vi "ScanAction.vi"(8 "error in (no error)":errorcluster caption="entrée d'erreur (pas d'erreur)", 9 "IndicePoint":i32, 10 "Dir":bool, 11 "Tools In":refnum<class "AttoANC300.lvclass"> caption="DNL_LabVIEW Object in") -> (0 "error out":errorcluster caption="sortie d'erreur", 2 "ScanParsOut":dbl[](array[numeric]), 3 "Tools Out":refnum<class "AttoANC300.lvclass"> caption="DNL_LabVIEW Object out")   [LabVIEW 2019, in "AttoANC300.lvclass"]
uses:
  AttoANC300.lvclass
  C:/Programmes Labview/LabscanV1A/DevicesClass/BaseDevice/BaseDevice.lvclass
  AttoANC300.lvclass/AttoANC300.ctl
  AttoAMC/ScanActionStates.ctl
  <userlib>/GenProg/WritebyWeakRefNum.vi
  <vilib>/Utility/error.llb/Error Cluster From Error Code.vi
  <vilib>/ErrorRing/Error Ring.xnode
  <userlib>/AMC300/AMC_VIs.lvlib
panel:
  in  "Reactivate":bool
  out "axis":i32
  out "Bkwd":bool
  out "Fwd":bool
  out "Trgt Rng(nm)":dbl
  in  "CtrlLpReact":u32
  out "PosDiff(nm)":dbl
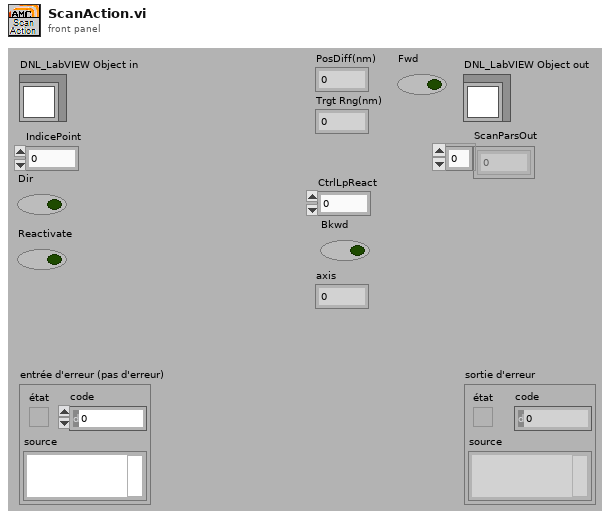
[diagram p1: front panel]
types:
  T1 = typedef "ScanActionStates.ctl" = enum16{"ReadPosDiff", "SetTarget", "WaitMoveDone", "MoveDone", "Timeout", "Ctrl_Loop_React", "Limit_check", "Error"}
  T2 = typedef "AttoANC300.lvclass/AttoANC300_Func.ctl" = enum16{"MotionMon (um)", "VoltDC (V)"}
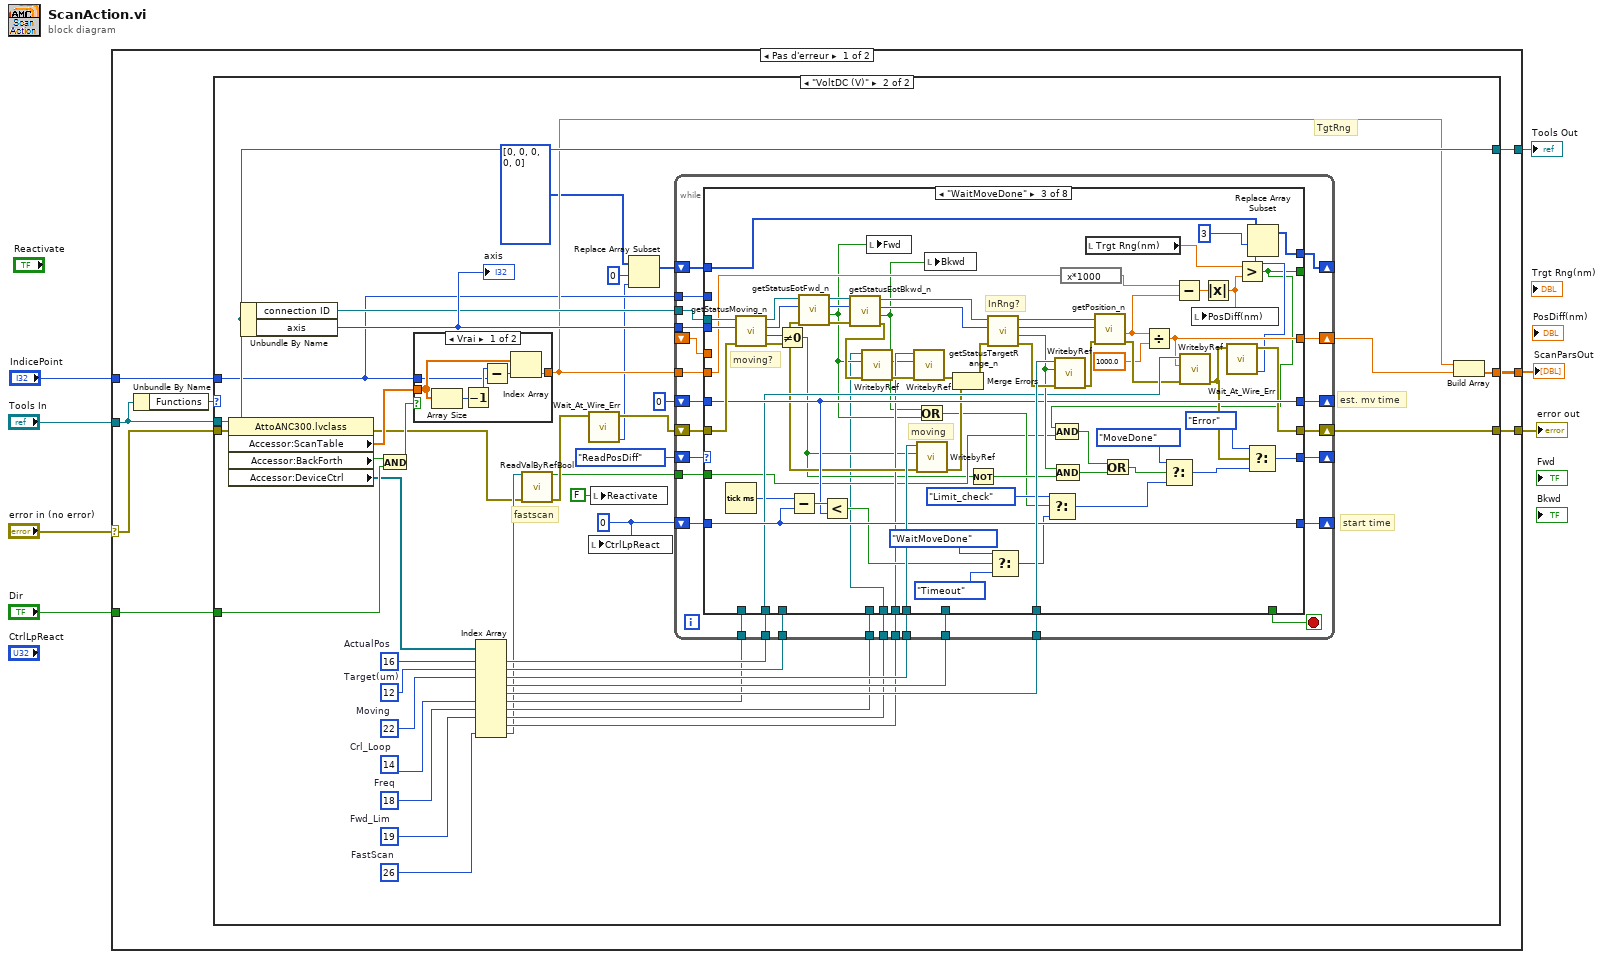
[diagram p0: block diagram]
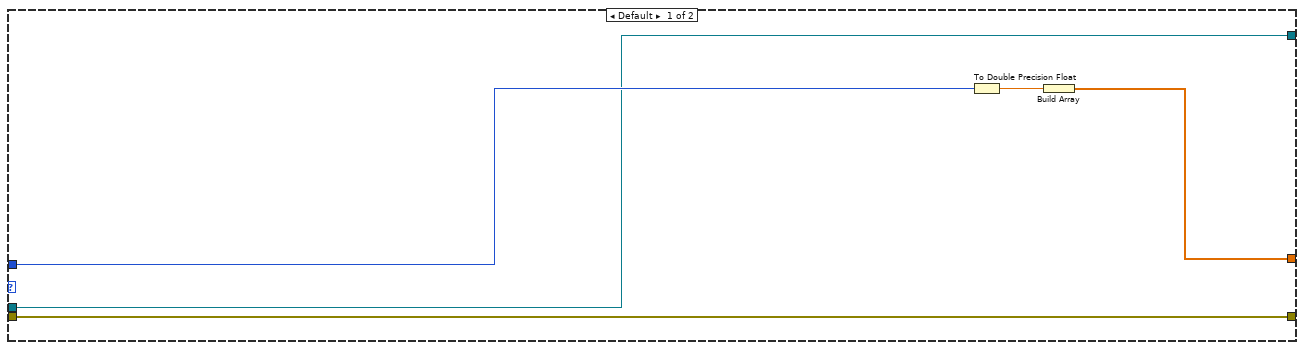
[diagram p2: hidden frame]
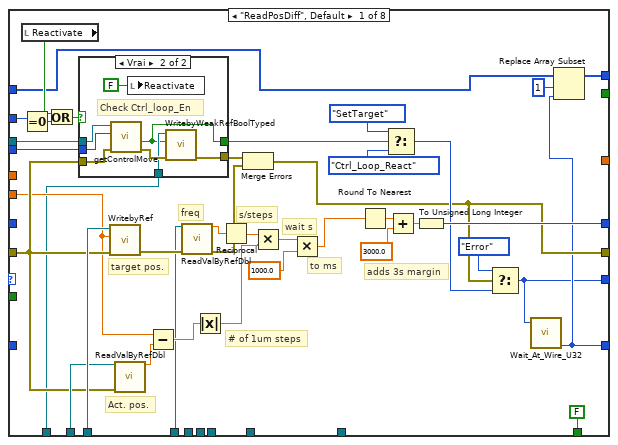
[diagram p3: hidden frame]
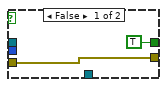
[diagram p4: hidden frame]
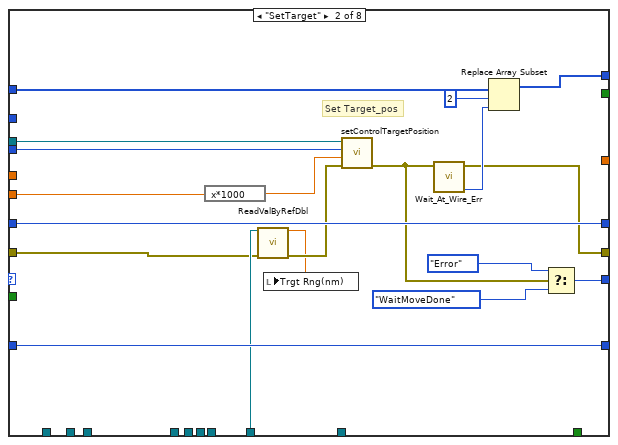
[diagram p5: hidden frame]
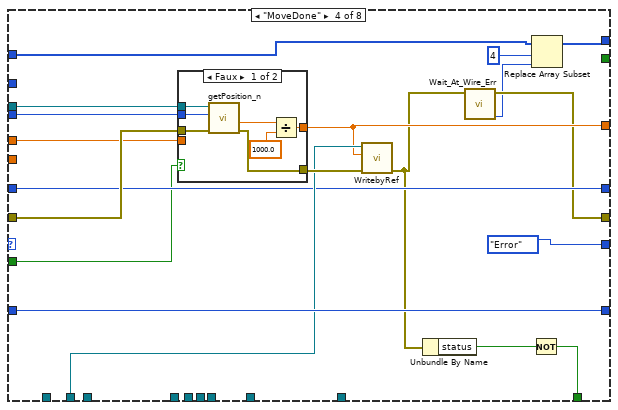
[diagram p6: hidden frame]
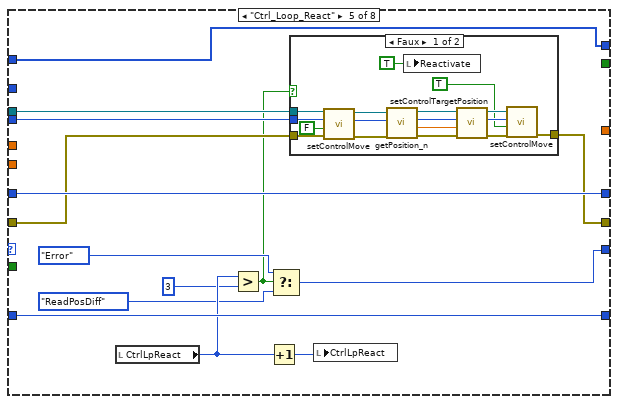
[diagram p8: hidden frame]
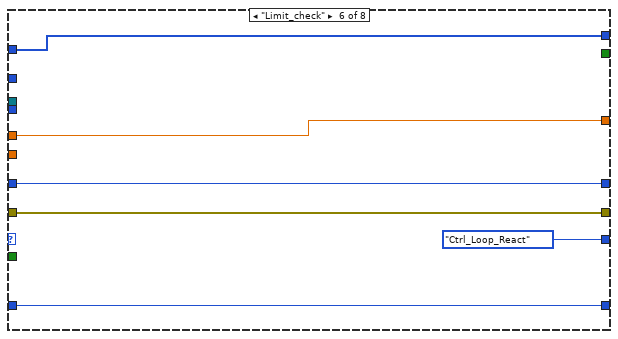
[diagram p10: hidden frame]
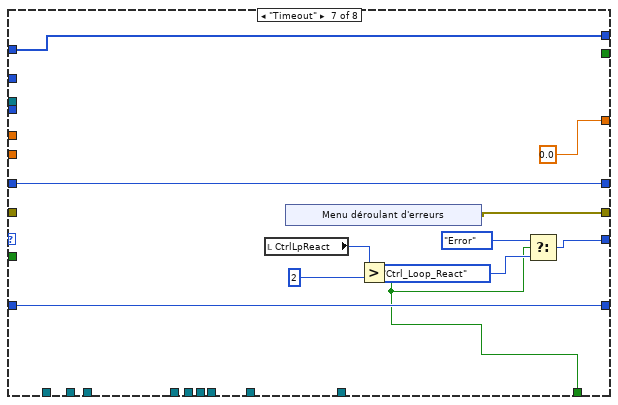
[diagram p11: hidden frame]
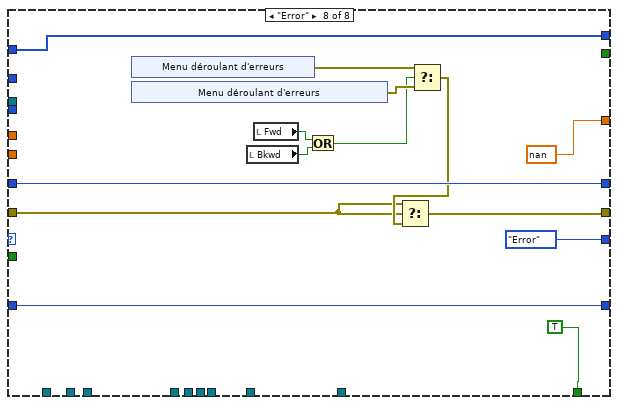
[diagram p12: hidden frame]
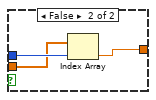
[diagram p13: hidden frame]
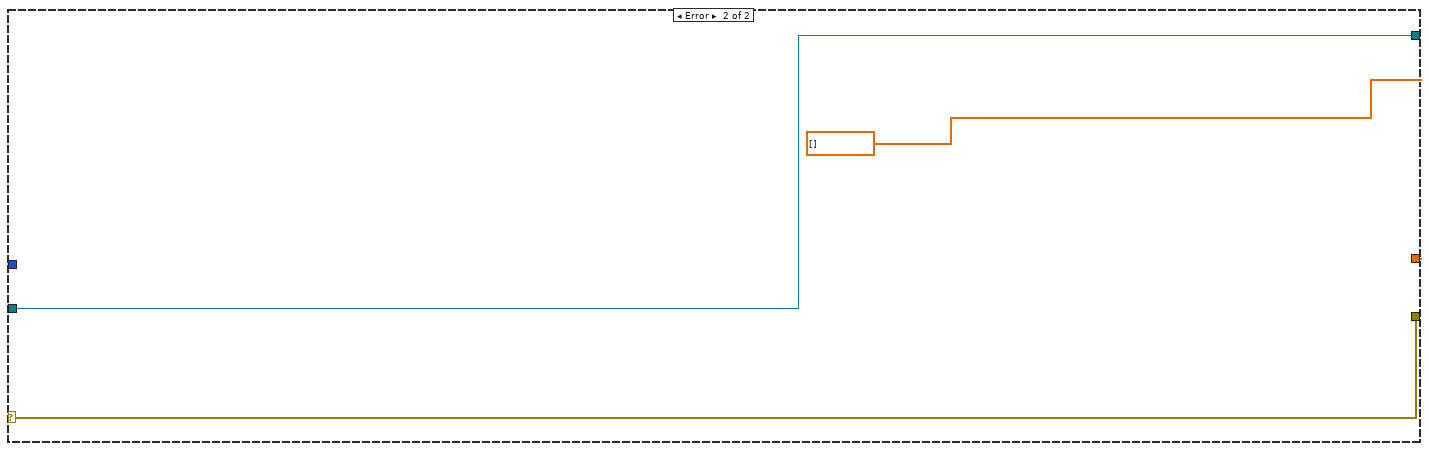
[diagram p14: hidden frame]
diagram:
  n1 = case shown="Pas d'erreur" "error in (no error)" {
    selector: "error in (no error)" -> [w12 w342]
    tunnel: "Tools In" -> [w13 w341]
    tunnel: [w11 dbl[] []] -> w2
    tunnel: [w10 w342] -> w5
    tunnel: [w9 w341] -> w4
    tunnel: "IndicePoint" -> [w14 _]
    tunnel: "Dir" -> [w8 _]
    frame No Error {
      n2 = Unbundle By Name(w13) -> ("Functions"=w15:T2)
      n3 = case shown="\"VoltDC (V)\"" w15 {
        tunnel: [w16 w63] -> w11
        tunnel: w14 -> [w20 w29]
        tunnel: [w18 w62] -> w9
        tunnel: w13 -> [w18 w62]
        tunnel: w12 -> [w17 w61]
        tunnel: [w17 w49] -> w10
        tunnel: w8 -> [_ w57]
        frame Default {
          n4 = To Double Precision Float(number=w20) -> (double precision float=w19:dbl)
          n5 = Build Array(w19) -> (w16:dbl[])
        }
        frame "VoltDC (V)" {
          w26 = u32 0 ("millisecond timer value")
          w34 = 26  # FastScan
          w39 = 19  # Fwd_Lim
          w41 = 18  # Freq
          w43 = 14  # Crl_Loop
          w51 = 12  # Target(um)
          w54 = 22  # Moving
          w55 = 16  # ActualPos
          # "est. mv time"
          # "start time"
          # "fastscan"
          # "TgtRng"
          n6 = property class="AttoANC300.lvclass"(reference=w62, error in=w61) -> (error out=w32:errorcluster, "Accessor:ScanTable"=w60:dbl[], "Accessor:BackForth"=w59:bool, "Accessor:DeviceCtrl"=w56:refnum<vi>[])  [unwired: 1 out]
          n7 = Unbundle By Name(w62) -> ("connection ID"=w47:refnum<k5>, "axis"=w48:i32)
          "axis" <- w48
          n8 = And(x=w59, y=w57) -> (x .and. y?=w58:bool)
          n9 = case shown="Vrai" w58 {
            tunnel: w29 -> [w331 w339]
            tunnel: [w336 w337] -> w36
            tunnel: w60 -> [w335 w338]
            frame True {
              n10 = Array Size(array=w335) -> (size(s)=w334:i32)
              n11 = Decrement(x=w334) -> (x-1=w332:i32)
              n12 = Subtract(x=w332, y=w331) -> (x-y=w333:i32)
              n13 = Index Array(array=w335, index=w333) -> (element=w336:dbl)
            }
            frame False {
              n14 = Index Array(array=w338, index=w339) -> (element=w337:dbl)
            }
          }
          n15 = Index Array(array=w56, index #1=w55, index #2=w51, index #3=w54, index #6=w43, index #7=w41, index #8=w39, index #10=w34) -> (element #1=w46:refnum<vi>, element #2=w52:refnum<vi>, element #3=w53:refnum<vi>, element #4=w44:refnum<vi>, element #5=w45:refnum<vi>, element #6=w42:refnum<vi>, element #7=w40:refnum<vi>, element #8=w38:refnum<vi>, element #9=w37:refnum<vi>, element #10=w33:refnum<vi>)  [unwired: 3 in]
          n16 = call <userlib>:"ReadValByRefBool.vi"("Control Ref"=w33, "error in"=w32) -> ("Valeur"=w30:bool, "error out"=w31:errorcluster)  [unwired: 12 in]
          n17 = call <userlib>:"Wait_At_Wire_Err.vi"("error in (no error)"=w31) -> ("Clock(ms)"=w22:u32, "error out"=w25:errorcluster)  [unwired: 8 in, 1 out]
          n18 = local write "CtrlLpReact"(w26) -> ()
          n19 = local write "Reactivate"(FALSE ("Reactivate")) -> ()
          n20 = Replace Array Subset(array=u32[] [0, 0, 0, 0, 0] ("Clock(ms)"), new element=w22, index=0 ("indice")) -> (w24:u32[])
          n21 = while {
            tunnel: w53 -> [w90]
            tunnel: w52 -> [w89]
            tunnel: w45 -> [w87]
            tunnel: w48 -> [w85]
            tunnel: w47 -> [w84]
            tunnel: w46 -> [w82]
            shift-right: [w86] -> w49
            shift-left: w25 -> [w83]
            shift-right: [w79] -> _
            shift-left: w26 -> [w76]
            shift-right: [w78] -> _
            shift-left: ScanActionStates."ReadPosDiff" -> [w80]
            shift-right: [w75] -> _
            shift-left: u32 0 -> [w74]
            tunnel: w44 -> [w73]
            tunnel: w42 -> [w72]
            tunnel: w40 -> [w71]
            tunnel: w38 -> [w70]
            tunnel: w37 -> [w69]
            tunnel: w36 -> [w81]
            shift-right: [w68] -> _
            shift-left: w24 -> [w67]
            tunnel: w30 -> [w66]
            tunnel: w29 -> [w65]
            shift-right: [w88] -> w50
            shift-left: _ -> [w64]
            stop <- w77 stop-if-true
            n22 = case shown="\"WaitMoveDone\"" w80 {
              tunnel: w90 -> [_ _ w224 _ _ _ _ _]
              tunnel: w89 -> [w129 _ _ _ _ _ _ _]
              tunnel: [_ _ w180 w237 _ w285 0.0 ("ScanParamIn") nan ("ScanParamIn")] -> w88
              tunnel: w87 -> [_ _ w223 _ _ _ _ _]
              tunnel: [w108 w140 w168 w231 w255 w288 w298 w308] -> w86
              tunnel: w85 -> [w116 w150 w220 w239 w263 _ _ _]
              tunnel: w84 -> [w117 w151 w221 w240 w264 _ _ _]
              tunnel: w83 -> [w115 w152 w219 w238 w262 w288 _ w309]
              tunnel: w82 -> [w125 _ w205 w241 _ _ _ _]
              tunnel: w81 -> [w107 w148 w179 _ _ _ _ _]
              tunnel: [w95 w156 w218 w242 w265 w289 w301 w318] -> w79
              tunnel: [w94 w157 w209 ScanActionStates."Error" w256 ScanActionStates."Ctrl_Loop_React" w292 ScanActionStates."Error"] -> w78
              tunnel: [FALSE _ _ w234 _ _ w293 TRUE] -> w77
              tunnel: w76 -> [_ w156 w218 w242 w265 w289 w301 w318]
              tunnel: [w121 w155 w215 w236 w266 w290 w300 w317] -> w75
              tunnel: w74 -> [_ w155 w215 w236 w266 w290 w300 w317]
              tunnel: w73 -> [_ w153 _ _ _ _ _ _]
              tunnel: [_ _ w163 _ _ _ _ _] -> _
              tunnel: w72 -> [w98 _ _ _ _ _ _ _]
              tunnel: w71 -> [w119 _ _ _ _ _ _ _]
              tunnel: w70 -> [_ _ w159 _ _ _ _ _]
              tunnel: w69 -> [_ _ w193 _ _ _ _ _]
              tunnel: [w100 w143 w172 w227 w253 w286 w291 w307] -> w68
              tunnel: w67 -> [w91 w144 w171 w228 w253 w286 w291 w307]
              tunnel: w66 -> [_ _ w164 w225 _ _ _ _]
              tunnel: w65 -> [w97 _ _ _ _ _ _ _]
              tunnel: w64 -> [_ _ _ w226 _ w285 _ _]
              frame "ReadPosDiff", Default {
                # "adds 3s margin"
                # "to ms"
                # "freq"
                # "s/steps"
                # "wait s"
                # "# of 1um steps"
                # "Act. pos."
                # "target pos."
                n23 = local read "Reactivate"() -> (w92:bool)
                n24 = Equal To 0?(x=w97) -> (x = 0?=w96:bool)
                n25 = Or(x=w92, y=w96) -> (x .or. y?=w93:bool)
                n26 = case shown="Vrai" w93 {
                  tunnel: w117 -> [_ w139]
                  tunnel: w116 -> [_ w138]
                  tunnel: w115 -> [w131 w133]
                  tunnel: [w131 w136] -> w113
                  tunnel: [TRUE ("controll move out") w134] -> w109
                  tunnel: w98 -> [_ w135]
                  frame False {
                  }
                  frame True {
                    # "Check Ctrl_loop_En"
                    n27 = call <userlib>:"getControlMove.vi"("error in"=w133, "axis"=w138, "connection ID"=w139) -> ("error out"=w137:errorcluster, "enable"=w134:bool)  [unwired: 5 in, 2 out]
                    n28 = local write "Reactivate"(FALSE ("Reactivate")) -> ()
                    n29 = call <userlib>:"WritebyWeakRefBoolTyped.vi"("error in"=w137, "Valeur"=w134, "Control Ref"=w135) -> ("error out"=w136:errorcluster)  [unwired: 8 in]
                  }
                }
                n30 = call-poly <userlib>:"WritebyRef.vi"("error in"=w115, "Valeur"=w107, "Control Ref"=w129) -> ("error out"=w120:errorcluster)  [unwired: 8 in]
                n31 = call <userlib>:"ReadValByRefDbl.vi"("Control Ref"=w125, "error in"=w115) -> ("Valeur"=w128:dbl)  [unwired: 12 in, 1 out]
                n32 = Subtract(x=w107, y=w128) -> (x-y=w127:dbl)
                n33 = call <userlib>:"ReadValByRefDbl.vi"("Control Ref"=w119, "error in"=w120) -> ("Valeur"=w118:dbl, "error out"=w114:errorcluster)  [unwired: 12 in]
                n34 = Absolute Value(x=w127) -> (abs(x)=w104:dbl)
                n35 = Reciprocal(x=w118) -> (1/x=w126:dbl)
                n36 = Merge Errors(w113, w114) -> (w108:errorcluster)
                n37 = Multiply(x=w126, y=w104) -> (x*y=w103:dbl)
                n38 = Multiply(x=w103, y=1000.0) -> (x*y=w102:dbl)
                n39 = Round To Nearest(number=w102) -> (nearest integer value=w122:dbl)
                n40 = Select(t=ScanActionStates."SetTarget", s=w109, f=ScanActionStates."Ctrl_Loop_React") -> (s? t:f=w112:T1)
                n41 = Add(x=w122, y=3000.0) -> (x+y=w106:dbl)
                n42 = To Unsigned Long Integer(number=w106) -> (unsigned 32bit integer=w121:u32)
                n43 = Select(t=ScanActionStates."Error", s=w108, f=w112) -> (s? t:f=w94:T1)
                n44 = call <userlib>:"Wait_At_Wire_U32.vi"("error in (no error)"=w94) -> ("Clock(ms)"=w95:u32)  [unwired: 8 in, 2 out]
                n45 = Replace Array Subset(array=w91, new element=w95, index=1 ("indice")) -> (w100:u32[])
              }
              frame "SetTarget" {
                # "Set Target_pos"
                n46 = expression code="x*1000"(w148) -> (w147:dbl)
                n47 = call <userlib>:"ReadValByRefDbl.vi"("Control Ref"=w153, "error in"=w152) -> ("Valeur"=w146:dbl, "error out"=w154:errorcluster)  [unwired: 12 in]
                n48 = local write "Trgt Rng(nm)"(w146) -> ()
                n49 = call <userlib>:"setControlTargetPosition.vi"("error in"=w154, "target"=w147, "axis"=w150, "connection ID"=w151) -> ("error out"=w145:errorcluster)  [unwired: 5 in, 2 out]
                n50 = call <userlib>:"Wait_At_Wire_Err.vi"("error in (no error)"=w145) -> ("Clock(ms)"=w141:u32, "error out"=w140:errorcluster)  [unwired: 8 in, 1 out]
                n51 = Replace Array Subset(array=w144, new element=w141, index=2 ("indice")) -> (w143:u32[])
                n52 = Select(t=ScanActionStates."Error", s=w145, f=ScanActionStates."WaitMoveDone") -> (s? t:f=w157:T1)
              }
              frame "WaitMoveDone" {
                # "moving"
                # "InRng?"
                # "moving?"
                n53 = Tick Count (ms)() -> (millisecond timer value=w173:u32)
                n54 = call <userlib>:"getStatusMoving_n.vi"("error in"=w219, "axis"=w220, "connection ID"=w221) -> ("error out"=w195:errorcluster, "status"=w161:i32, "axis_out"=w199:i32, "connection ID"=w200:refnum<k5>)  [unwired: 5 in]
                n55 = Not Equal To 0?(x=w161) -> (x != 0?=w160:bool)
                n56 = Subtract(x=w173, y=w218) -> (x-y=w216:u32)
                n57 = call <userlib>:"getStatusEotFwd_n.vi"("error in"=w195, "axis"=w199, "connection ID"=w200) -> ("error out"=w202:errorcluster, "detected"=w174:bool, "axis_out"=w201:i32, "connection ID"=w198:refnum<k5>)  [unwired: 5 in]
                n58 = Less?(x=w216, y=w215) -> (x < y?=w212:bool)
                n59 = call <userlib>:"getStatusEotBkwd_n.vi"("error in"=w202, "axis"=w201, "connection ID"=w198) -> ("error out"=w192:errorcluster, "detected"=w175:bool, "axis_out"=w196:i32, "connection ID"=w197:refnum<k5>)  [unwired: 5 in]
                n60 = call-poly <userlib>:"WritebyRef.vi"("error in"=w192, "Valeur"=w174, "Control Ref"=w159) -> ("error out"=w194:errorcluster)  [unwired: 8 in]
                n61 = local write "Fwd"(w174) -> ()
                n62 = call-poly <userlib>:"WritebyRef.vi"("error in"=w194, "Valeur"=w175, "Control Ref"=w193) -> ("error out"=w189:errorcluster)  [unwired: 8 in]
                n63 = Or(x=w175, y=w174) -> (x .or. y?=w186:bool)
                n64 = call-poly <userlib>:"WritebyRef.vi"("error in"=w195, "Valeur"=w160, "Control Ref"=w224) -> ("error out"=w191:errorcluster)  [unwired: 8 in]
                n65 = local write "Bkwd"(w175) -> ()
                n66 = Merge Errors(w189, w191) -> (w190:errorcluster)
                n67 = Not(x=w160) -> (.not. x?=w188:bool)
                n68 = call <userlib>:"getStatusTargetRange_n.vi"("error in"=w190, "axis"=w196, "connection ID"=w197) -> ("error out"=w222:errorcluster, "in_range"=w217:bool, "axis_out"=w207:i32, "connection ID"=w208:refnum<k5>)  [unwired: 5 in]
                n69 = Select(t=ScanActionStates."WaitMoveDone", s=w212, f=ScanActionStates."Timeout") -> (s? t:f=w183:T1)
                n70 = Select(t=ScanActionStates."Limit_check", s=w186, f=w183) -> (s? t:f=w184:T1)
                n71 = call-poly <userlib>:"WritebyRef.vi"("error in"=w222, "Valeur"=w217, "Control Ref"=w223) -> ("error out"=w206:errorcluster)  [unwired: 8 in]
                n72 = Compound Arithmetic op=AND(w217, w188) -> (w166:bool)
                n73 = expression code="x*1000"(w179) -> (w178:dbl)
                n74 = local read "Trgt Rng(nm)"() -> (w181:dbl)
                n75 = call <userlib>:"getPosition_n.vi"("error in"=w206, "axis"=w207, "connection ID"=w208) -> ("error out"=w177:errorcluster, "position"=w182:dbl)  [unwired: 5 in, 2 out]
                n76 = Divide(x=w182, y=1000.0 ("x")) -> (x/y=w180:dbl)
                n77 = Subtract(x=w178, y=w182) -> (x-y=w204:dbl)
                n78 = call-poly <userlib>:"WritebyRef.vi"("error in"=w177, "Valeur"=w180, "Control Ref"=w205) -> ("error out"=w169:errorcluster)  [unwired: 8 in]
                n79 = Absolute Value(x=w204) -> (abs(x)=w203:dbl)
                n80 = local write "PosDiff(nm)"(w203) -> ()
                n81 = call <userlib>:"Wait_At_Wire_Err.vi"("error in (no error)"=w169) -> ("Clock(ms)"=w167:u32, "error out"=w168:errorcluster)  [unwired: 8 in, 1 out]
                n82 = Greater?(x=w181, y=w203) -> (0:w163:bool)
                n83 = Compound Arithmetic op=AND(w163, w164) -> (w162:bool)
                n84 = Or(x=w162, y=w166) -> (x .or. y?=w165:bool)
                n85 = Select(t=ScanActionStates."MoveDone", s=w165, f=w184) -> (s? t:f=w213:T1)
                n86 = Select(t=ScanActionStates."Error", s=w169, f=w213) -> (s? t:f=w209:T1)
                n87 = Replace Array Subset(array=w171, new element=w167, index=3 ("indice")) -> (w172:u32[])
              }
              frame "MoveDone" {
                n88 = case shown="Faux" w225 {
                  tunnel: [w250 w252] -> w243
                  tunnel: w240 -> [w248 _]
                  tunnel: w239 -> [w247 _]
                  tunnel: w238 -> [w246 w252]
                  tunnel: [w245 w251] -> w237
                  tunnel: w226 -> [_ w251]
                  frame False {
                    n89 = call <userlib>:"getPosition_n.vi"("error in"=w246, "axis"=w247, "connection ID"=w248) -> ("error out"=w250:errorcluster, "position"=w249:dbl)  [unwired: 5 in, 2 out]
                    n90 = Divide(x=w249, y=1000.0) -> (x/y=w245:dbl)
                  }
                  frame True {
                  }
                }
                n91 = call-poly <userlib>:"WritebyRef.vi"("error in"=w243, "Valeur"=w237, "Control Ref"=w241) -> ("error out"=w232:errorcluster)  [unwired: 8 in]
                n92 = Unbundle By Name(w232) -> ("status"=w235:bool)
                n93 = call <userlib>:"Wait_At_Wire_Err.vi"("error in (no error)"=w232) -> ("Clock(ms)"=w230:u32, "error out"=w231:errorcluster)  [unwired: 8 in, 1 out]
                n94 = Not(x=w235) -> (.not. x?=w234:bool)
                n95 = Replace Array Subset(array=w228, new element=w230, index=4 ("indice")) -> (w227:u32[])
              }
              frame "Ctrl_Loop_React" {
                n96 = local read "CtrlLpReact"() -> (w260:u32)
                n97 = Greater?(x=w260, y=u32 3) -> (0:w254:bool)
                n98 = Increment(x=w260) -> (x+1=w261:u32)
                n99 = Select(t=ScanActionStates."Error", s=w254, f=ScanActionStates."ReadPosDiff") -> (s? t:f=w256:T1)
                n100 = case shown="Faux" w254 {
                  tunnel: w264 -> [w275 _]
                  tunnel: w263 -> [w274 _]
                  tunnel: w262 -> [w273 w284]
                  tunnel: [w278 w284] -> w255
                  frame False {
                    n101 = call <userlib>:"setControlMove.vi"("error in"=w273, "enable"=FALSE ("control move in"), "axis"=w274, "connection ID"=w275) -> ("error out"=w272:errorcluster, "axis_out"=w270:i32, "connection ID"=w271:refnum<k5>)  [unwired: 5 in]
                    n102 = call <userlib>:"getPosition_n.vi"("error in"=w272, "axis"=w270, "connection ID"=w271) -> ("error out"=w280:errorcluster, "position"=w281:dbl, "axis_out"=w282:i32, "connection ID"=w283:refnum<k5>)  [unwired: 5 in]
                    n103 = local write "Reactivate"(TRUE ("Reactivate")) -> ()
                    n104 = call <userlib>:"setControlTargetPosition.vi"("error in"=w280, "target"=w281, "axis"=w282, "connection ID"=w283) -> ("error out"=w279:errorcluster, "axis_out"=w276:i32, "connection ID"=w277:refnum<k5>)  [unwired: 5 in]
                    n105 = call <userlib>:"setControlMove.vi"("error in"=w279, "enable"=TRUE ("Set"), "axis"=w276, "connection ID"=w277) -> ("error out"=w278:errorcluster)  [unwired: 5 in, 2 out]
                  }
                  frame True {
                  }
                }
                n106 = local write "CtrlLpReact"(w261) -> ()
              }
              frame "Limit_check" {
              }
              frame "Timeout" {
                n107 = local read "CtrlLpReact"() -> (w294:u32)
                n108 = xnode "Menu déroulant d'erreurs"() -> ("sortie d'erreur"=w298:errorcluster)
                n109 = Greater?(x=w294, y=u32 2) -> (0:w293:bool)
                n110 = Select(t=ScanActionStates."Error", s=w293, f=ScanActionStates."Ctrl_Loop_React") -> (s? t:f=w292:T1)
              }
              frame "Error" {
                n111 = xnode "Menu déroulant d'erreurs"() -> ("sortie d'erreur"=w315:errorcluster)
                n112 = xnode "Menu déroulant d'erreurs"() -> ("sortie d'erreur"=w314:errorcluster)
                n113 = local read "Bkwd"() -> (w312:bool)
                n114 = local read "Fwd"() -> (w313:bool)
                n115 = Or(x=w313, y=w312) -> (x .or. y?=w311:bool)
                n116 = Select(t=w315, s=w311, f=w314) -> (s? t:f=w310:errorcluster)
                n117 = Select(t=w309, s=w309, f=w310) -> (s? t:f=w308:errorcluster)
              }
            }
          }
          n118 = Build Array(w36, w50) -> (w63:dbl[])
        }
      }
    }
    frame Error {
    }
  }
  "error out" <- w5
  "Tools Out" <- w4
  "ScanParsOut" <- w2
